vi "Initiate Session.vi"(8 "error in (no error)":errorcluster, 11 "Driver in":refnum<class "Driver.lvclass">) -> (0 "error out":errorcluster, 3 "Driver out":refnum<class "Driver.lvclass">)   [LabVIEW 2023, in "HAF.lvlib" / "Driver.lvclass"]
doc: "Creates a Session for the Instrument that will be communicated with."
uses:
  Driver.lvclass
  Driver.lvclass/Driver.ctl
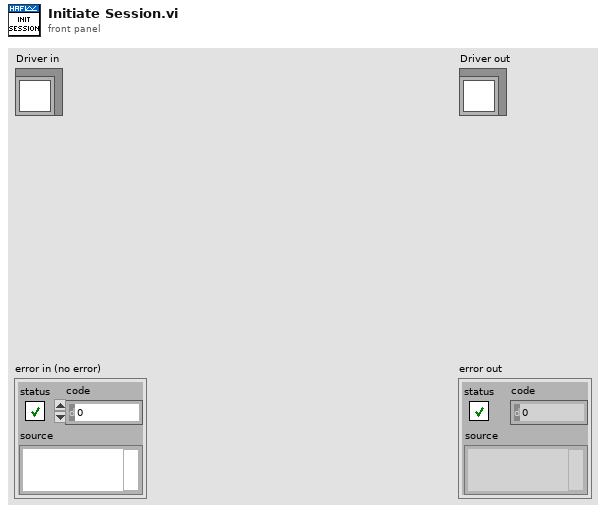
[diagram p1: front panel]
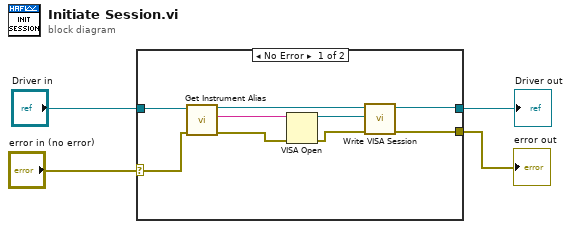
[diagram p0: block diagram]
diagram:
  n1 = case shown="No Error" "error in (no error)" {
    selector: "error in (no error)" -> [w12 w15]
    tunnel: [w5 w15] -> w3
    tunnel: [w6 w14] -> w1
    tunnel: "Driver in" -> [w13 w14]
    frame No Error {
      n2 = call-dynamic "Get Instrument Alias.vi"("error in (no error)"=w12, "Driver in"=w13) -> ("error out"=w10:errorcluster, "Instrument Alias"=w11:string, "Driver out"=w8:refnum<class "Driver.lvclass">)  [unwired: 7 in]
      n3 = VISA Open(error in (no error)=w10, VISA resource name=w11) -> (VISA resource name=w9:refnum<visa-resource-name>, error out=w7:errorcluster)  [unwired: 3 in]
      n4 = call-dynamic "Write VISA Session.vi"("error in (no error)"=w7, "VISA Session"=w9, "Driver in"=w8) -> ("error out"=w5:errorcluster, "Driver out"=w6:refnum<class "Driver.lvclass">)  [unwired: 7 in]
    }
    frame Error {
    }
  }
  "error out" <- w3
  "Driver out" <- w1
